vi "Load_Parsing.vi"(9 "ERD String Data in":string[](array[string]), 10 "Data":string, 11 "ERD_Always Show in":T1) -> (2 "ERD String Data out":string[](array[string]), 3 "ERD_Always Show out":T1)   [LabVIEW 2016]
uses:
  type defs2/ERD_Always_Show_Brass.ctl
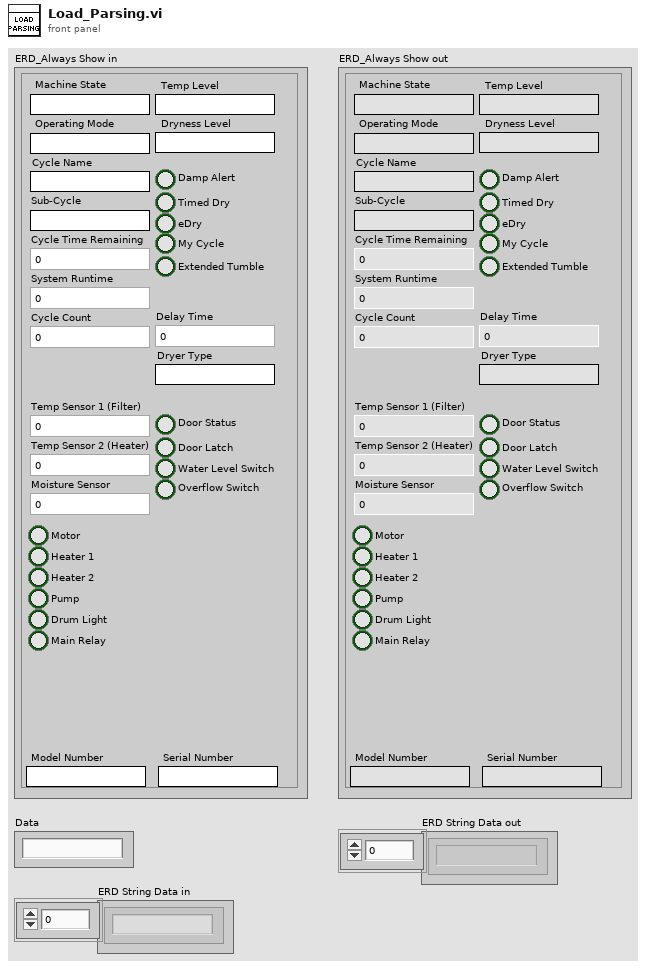
[diagram p1: front panel]
types:
  T1 = typedef "ERD_Always_Show_Brass.ctl" = cluster{"Machine State":string, "Cycle Count":u32, "Dryness Level":string, "Temp Level":string, "Delay Time":u16, "Sub-Cycle":string, "Cycle Name":string, "Model Number":string, "Serial Number":string, "System Runtime":u32, "Cycle Time Remaining":u16, "Operating Mode":string, "Temp Sensor 1 (Filter)":u16, "Water Level Switch":bool, "Overflow Switch":bool, "Door Status":bool, "Door Latch":bool, "Heater 1":bool, "Temp Sensor 2 (Heater)":u16, "Moisture Sensor":u16, "Dryer Type":string, "eDry":bool, "Damp Alert":bool, "Timed Dry":bool, "My Cycle":bool, "Extended Tumble":bool, "Heater 2":bool, "Pump":bool, "Drum Light":bool, "Main Relay":bool, "Motor":bool}
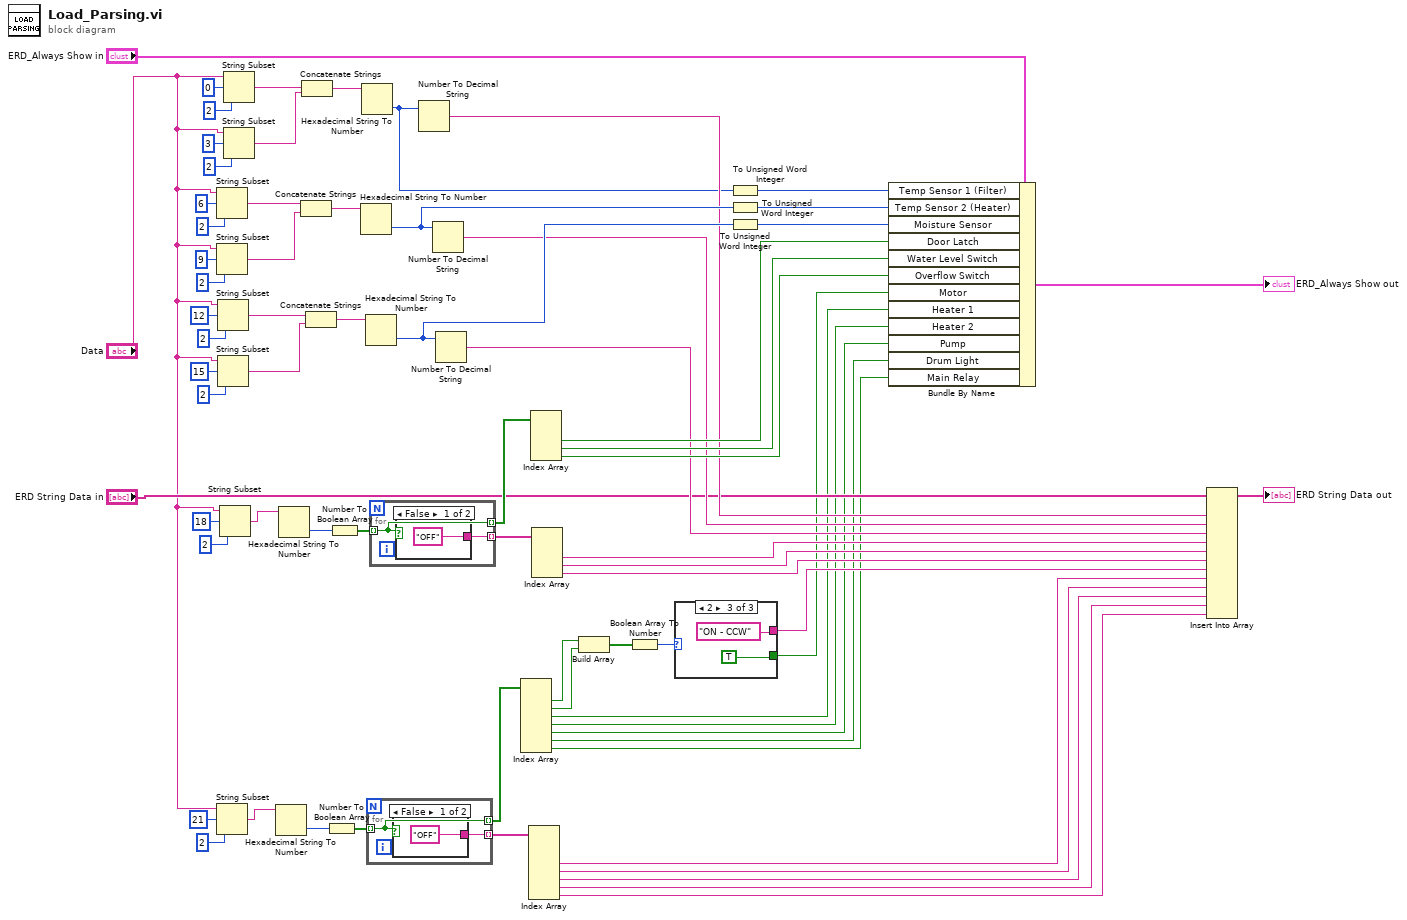
[diagram p0: block diagram]
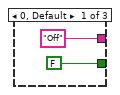
[diagram p2: hidden frame]
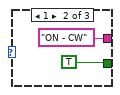
[diagram p3: hidden frame]
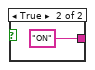
[diagram p4: hidden frame]
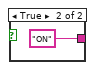
[diagram p5: hidden frame]
diagram:
  n1 = String Subset(string="Data", offset (0)=6, length (rest)=2 ("length (rest)")) -> (substring=w28:string)
  n2 = String Subset(string="Data", offset (0)=9, length (rest)=2 ("length (rest)")) -> (substring=w27:string)
  n3 = String Subset(string="Data", offset (0)=21, length (rest)=2 ("length (rest)")) -> (substring=w21:string)
  n4 = String Subset(string="Data", offset (0)=12, length (rest)=2 ("length (rest)")) -> (substring=w26:string)
  n5 = String Subset(string="Data", offset (0)=15, length (rest)=2 ("length (rest)")) -> (substring=w25:string)
  n6 = String Subset(string="Data", offset (0)=18, length (rest)=2 ("length (rest)")) -> (substring=w59:string)
  n7 = String Subset(string="Data", offset (0)=0, length (rest)=2 ("length (rest)")) -> (substring=w29:string)
  n8 = String Subset(string="Data", offset (0)=3, length (rest)=2 ("length (rest)")) -> (substring=w30:string)
  n9 = Hexadecimal String To Number(string=w21) -> (number=w22:u32)  [unwired: 2 in, 1 out]
  n10 = Hexadecimal String To Number(string=w59) -> (number=w60:u32)  [unwired: 2 in, 1 out]
  n11 = Concatenate Strings(w28, w27) -> (w48:string)
  n12 = Concatenate Strings(w29, w30) -> (w47:string)
  n13 = Concatenate Strings(w26, w25) -> (w49:string)
  n14 = Number To Boolean Array(number=w22) -> (Boolean array=w23:bool[])
  n15 = Number To Boolean Array(number=w60) -> (Boolean array=w63:bool[])
  n16 = Hexadecimal String To Number(string=w48) -> (number=w61:u32)  [unwired: 2 in, 1 out]
  n17 = Hexadecimal String To Number(string=w47) -> (number=w53:u32)  [unwired: 2 in, 1 out]
  n18 = Hexadecimal String To Number(string=w49) -> (number=w62:u32)  [unwired: 2 in, 1 out]
  n19 = for {
    tunnel: w23 -> [w73] mode=indexing
    tunnel: [w73] -> w17 mode=indexing
    tunnel: [w72] -> w24 mode=indexing
    n20 = case shown="False" w73 {
      tunnel: ["OFF" "ON"] -> w72
      frame False {
      }
      frame True {
      }
    }
  }
  n21 = for {
    tunnel: w63 -> [w77] mode=indexing
    tunnel: [w77] -> w65 mode=indexing
    tunnel: [w76] -> w64 mode=indexing
    n22 = case shown="False" w77 {
      tunnel: ["OFF" "ON"] -> w76
      frame False {
      }
      frame True {
      }
    }
  }
  n23 = Number To Decimal String(number=w53) -> (decimal integer string=w54:string)  [unwired: 1 in]
  n24 = Number To Decimal String(number=w61) -> (decimal integer string=w55:string)  [unwired: 1 in]
  n25 = Number To Decimal String(number=w62) -> (decimal integer string=w56:string)  [unwired: 1 in]
  n26 = Index Array(array=w17) -> (element #1=w16:bool, element #2=w15:bool, element #3=w5:bool, element #4=w4:bool, element #5=w3:bool, element #6=w2:bool, element #7=w1:bool)  [unwired: 7 in]
  n27 = Index Array(array=w24) -> (element #3=w10:string, element #4=w9:string, element #5=w8:string, element #6=w7:string, element #7=w6:string)  [unwired: 7 in, 2 out]
  n28 = Index Array(array=w65) -> (element #2=w71:bool, element #3=w70:bool, element #4=w69:bool)  [unwired: 4 in, 1 out]
  n29 = Index Array(array=w64) -> (element #2=w68:string, element #3=w67:string, element #4=w66:string)  [unwired: 4 in, 1 out]
  n30 = Build Array(w16, w15) -> (w14:bool[])
  n31 = Boolean Array To Number(Boolean array=w14) -> (number=w13:u32)
  n32 = case shown="2" w13 {
    tunnel: ["Off" "ON - CW" "ON - CCW"] -> w12
    tunnel: [FALSE TRUE TRUE] -> w11
    frame 0, Default {
    }
    frame 1 {
    }
    frame 2 {
    }
  }
  n33 = To Unsigned Word Integer(number=w53) -> (unsigned 16bit integer=w52:u16)
  n34 = To Unsigned Word Integer(number=w61) -> (unsigned 16bit integer=w51:u16)
  n35 = To Unsigned Word Integer(number=w62) -> (unsigned 16bit integer=w50:u16)
  n36 = Bundle By Name(cluster="ERD_Always Show in", "Temp Sensor 1 (Filter)"=w52, "Temp Sensor 2 (Heater)"=w51, "Moisture Sensor"=w50, "Door Latch"=w71, "Water Level Switch"=w70, "Overflow Switch"=w69, "Motor"=w11, "Heater 1"=w5, "Heater 2"=w4, "Pump"=w3, "Drum Light"=w2, "Main Relay"=w1) -> (→"ERD_Always Show out":T1)
  n37 = Insert Into Array(array="ERD String Data in", new element #1=w54, new element #2=w55, new element #3=w56, new element #4=w68, new element #5=w67, new element #6=w66, new element #7=w12, new element #8=w10, new element #9=w9, new element #10=w8, new element #11=w7, new element #12=w6) -> (→"ERD String Data out":string[])  [unwired: 1 in]
